vi "SettingChannels.GetRefs.vi"(8 "error in (no error)":errorcluster, 11 "Item Ref in":T1 format="%.0x") -> (0 "error out":errorcluster, 2 "Settings":T1[](array[typedef]) format="%.0x", 3 "Section Ref out":T1 format="%.0x")   [LabVIEW 2019, in "Diagnostics Addon System Explorer.lvlib"]
uses:
  Diagnostics Addon System Explorer.lvlib
  <vilib>/NI VeriStand/Custom Device API/Custom Device Item Ref.ctl
  Shared/SubVIs/Constants.vi
  <vilib>/NI VeriStand/Custom Device Tools/Custom Device Utility Library/NI VeriStand - Search for Item by GUID.vi
  <vilib>/NI VeriStand/Custom Device Tools/Custom Device Utility Library/Custom Device Utility Library.lvlib
  Shared/Diagnostics Addon Shared.lvlib
  <vilib>/NI VeriStand/Custom Device API/Custom Device API.lvlib
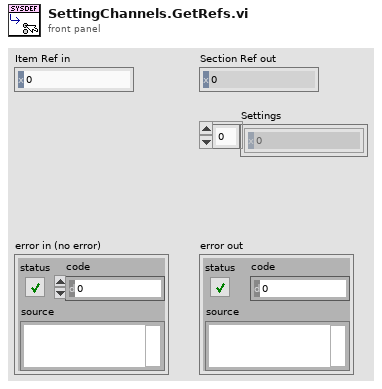
[diagram p1: front panel]
types:
  T1 = typedef "Custom Device API.lvlib/Custom Device Item Ref.ctl" = u64
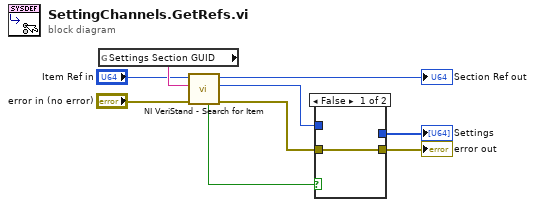
[diagram p0: block diagram]
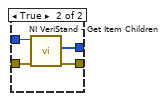
[diagram p2: hidden frame]
diagram:
  n1 = global read "Constants.vi" "Settings Section GUID"() -> (w9:string)
  n2 = call-poly <vilib>:"NI VeriStand - Search for Item.vi"("error in"="error in (no error)", "Item GUID"=w9, "Section Ref in"="Item Ref in") -> ("error out"=w4:errorcluster, "Item Ref"=w5:T1, "Section Ref out"=→"Section Ref out":T1, "Found"=w2:bool)  [unwired: 5 in]
  n3 = case shown="False" w2 {
    tunnel: w5 -> [_ w14]
    tunnel: w4 -> [w10 w13]
    tunnel: [w10 w12] -> w3
    tunnel: [_ w11] -> w1
    frame False {
    }
    frame True {
      n4 = call <vilib>:"NI VeriStand - Get Item Children.vi"("error in (no error)"=w13, "Item Ref in"=w14) -> ("error out"=w12:errorcluster, "Child Refs"=w11:T1[])  [unwired: 6 in, 2 out]
    }
  }
  "Settings" <- w1
  "error out" <- w3
